vi "Add WfmGraph Section.vi"(7 "Waveform Graph":refnum<vi>, 8 "error in":errorcluster, 11 "File refnum in":refnum<file>) -> (0 "error out":errorcluster, 3 "File refnum out":refnum<file>)   [LabVIEW 2021]
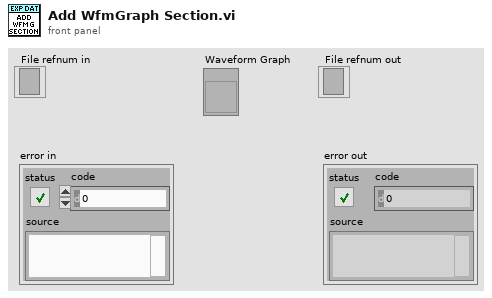
[diagram p1: front panel]
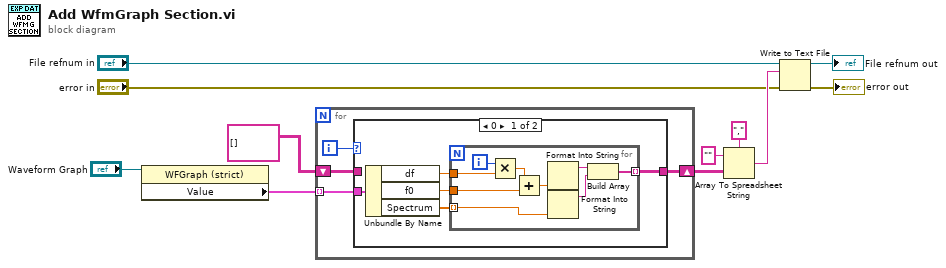
[diagram p0: block diagram]
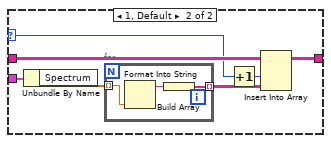
[diagram p2: hidden frame]
diagram:
  n1 = property class="WFGraph (strict)"(reference="Waveform Graph") -> ("Value"=w5:cluster{"f0":dbl, "df":dbl, "Spectrum":dbl[]}[])  [unwired: 1 in, 2 out]
  n2 = for {
    tunnel: w5 -> [w15] mode=indexing
    shift-right: [w14] -> w7
    shift-left: string[][] [] -> [w12]
    i -> [w13]
    n3 = case shown="0" w13 {
      selector: w13 -> [_ w31]
      tunnel: w15 -> [w17 w35]
      tunnel: [w16 w32] -> w14
      tunnel: w12 -> [_ w34]
      frame 0 {
        n4 = Unbundle By Name(w17) -> ("df"=w19:dbl, "f0"=w20:dbl, "Spectrum"=w18:dbl[])
        n5 = for {
          tunnel: w18 -> [w24] mode=indexing
          tunnel: w19 -> [w28]
          tunnel: w20 -> [w26]
          tunnel: [w22] -> w16 mode=indexing
          i -> [w29]
          n6 = Multiply(x=w29, y=w28) -> (x*y=w27:dbl)
          n7 = Add(x=w27, y=w26) -> (x+y=w25:dbl)
          n8 = Format Into String(w25) -> (resulting string=w23:string)  [unwired: 3 in, 1 out]
          n9 = Format Into String(w24) -> (resulting string=w21:string)  [unwired: 3 in, 1 out]
          n10 = Build Array(w23, w21) -> (w22:string[])
        }
      }
      frame 1, Default {
        n11 = Unbundle By Name(w35) -> ("Spectrum"=w36:dbl[])
        n12 = for {
          tunnel: w36 -> [w39] mode=indexing
          tunnel: [w37] -> w33 mode=indexing
          n13 = Format Into String(w39) -> (resulting string=w38:string)  [unwired: 3 in, 1 out]
          n14 = Build Array(w38) -> (w37:string[])
        }
        n15 = Increment(x=w31) -> (x+1=w30:i32)
        n16 = Insert Into Array(array=w34, index (col)=w30, new element=w33) -> (w32:string[][])  [unwired: 1 in]
      }
    }
  }
  n17 = Array To Spreadsheet String(delimiter (Tab)=",", array=w7, 3:"" ("format string")) -> (spreadsheet string=w9:string)
  n18 = Write to Text File(file (use dialog)="File refnum in", text=w9, error in="error in") -> (refnum out=→"File refnum out":refnum<file>, error out=→"error out":errorcluster)  [unwired: 1 in, 1 out]
